vi "Convert Hex String to ASCII Hex.vi"(0 "“十六进制显示”字符串":string) -> (3 "“正常显示”字符串":string)   [LabVIEW 2012]
panel:
  # "注意：点击“右健”，\n可以看到：十六进制显示"
  # "注意：点击“右健”，\n可以看到：正常显示"
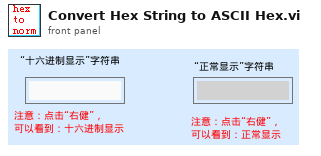
[diagram p1: front panel]
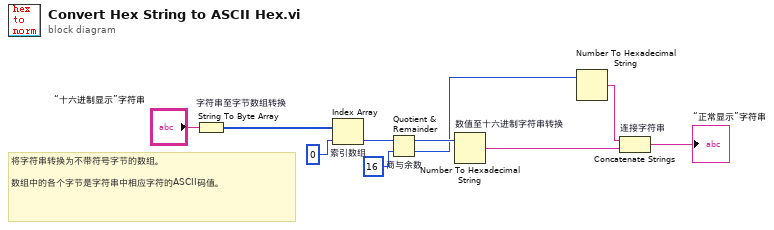
[diagram p0: block diagram]
diagram:
  # "将字符串转换为不带符号字节的数组。\n\n数组中的各个字节是字符串中相应字符的ASCII码值。"
  n1 = String To Byte Array "字符串至字节数组转换"(string="“十六进制显示”字符串") -> (unsigned byte array=w10:u8[])
  n2 = Index Array "索引数组"(array=w10, index=0) -> (element=w2:u8)
  n3 = Quotient & Remainder "商与余数"(x=w2, y=u8 16) -> (x-y*floor(x/y)=w6:u8, floor(x/y)=w5:u8)
  n4 = Number To Hexadecimal String "数值至十六进制字符串转换"(2:w6) -> (0:w3:string)  [unwired: 1 out]
  n5 = Number To Hexadecimal String(2:w5) -> (0:w4:string)  [unwired: 1 out]
  n6 = Concatenate Strings "连接字符串"(w4, w3) -> (→"“正常显示”字符串":string)
